vi "Fault_ID_Parse_FL24_Dryer.vi"(8 "Enum":enum16{"Sequence", "Table"}(ring), 11 "Numeric":u32) -> (3 "String":string)   [LabVIEW 2016]
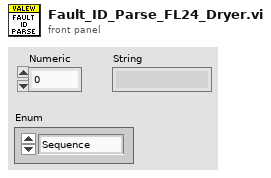
[diagram p1: front panel]
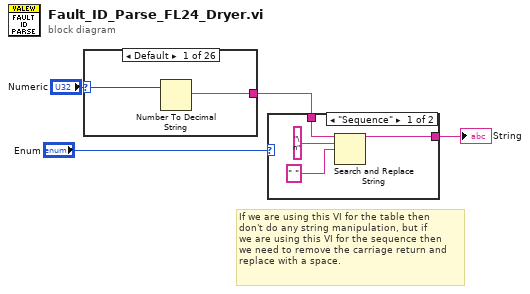
[diagram p0: block diagram]
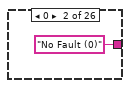
[diagram p3: hidden frame]
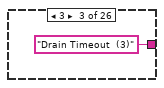
[diagram p4: hidden frame]
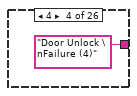
[diagram p5: hidden frame]
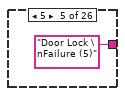
[diagram p6: hidden frame]
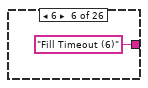
[diagram p7: hidden frame]
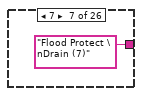
[diagram p8: hidden frame]
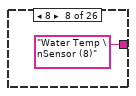
[diagram p9: hidden frame]
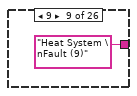
[diagram p10: hidden frame]
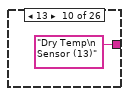
[diagram p11: hidden frame]
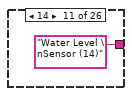
[diagram p12: hidden frame]
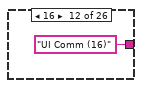
[diagram p13: hidden frame]
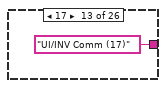
[diagram p14: hidden frame]
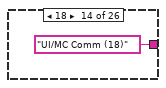
[diagram p15: hidden frame]
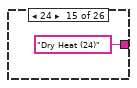
[diagram p16: hidden frame]
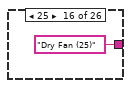
[diagram p17: hidden frame]
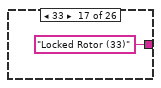
[diagram p18: hidden frame]
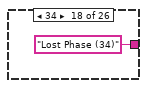
[diagram p19: hidden frame]
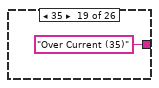
[diagram p20: hidden frame]
diagram:
  # "If we are using this VI for the table then\ndon't do any string manipulation, but if\nwe are using this VI for the sequence then\nwe need to remove the carriage return and\nreplace with a space."
  n1 = case shown="Default" "Numeric" {
    selector: "Numeric" -> [w6 _ _ _ _ _ _ _ _ _ _ _ _ _ _ _ _ _ _ _ _ _ _ _ _ _]
    tunnel: [w5 "No Fault (0)" "Drain Timeout  (3)" "Door Unlock \nFailure (4)" "Door Lock \nFailure (5)" "Fill Timeout (6)" "Flood Protect \nDrain (7)" "Water Temp \nSensor (8)" "Heat System \nFault (9)" "Dry Temp\n Sensor (13)" "Water Level \nSensor (14)" "UI Comm (16)" "UI/INV Comm (17)" "UI/MC Comm (18)" "Dry Heat (24)" "Dry Fan (25)" "Locked Rotor (33)" "Lost Phase (34)" "Over Current (35)" "Motor Current \nCircuit (36)" "Under \nVoltage (37)" "Motor \nOverheat (38)" "IMP Overheat (39)" "Drive Self \nCheck (40)" "MC Over \nVoltage (42)" "MC Check (43)"] -> w3
    frame Default {
      n2 = Number To Decimal String(number=w6) -> (decimal integer string=w5:string)  [unwired: 1 in]
    }
    frame 0 {
    }
    frame 3 {
    }
    frame 4 {
    }
    frame 5 {
    }
    frame 6 {
    }
    frame 7 {
    }
    frame 8 {
    }
    frame 9 {
    }
    frame 13 {
    }
    frame 14 {
    }
    frame 16 {
    }
    frame 17 {
    }
    frame 18 {
    }
    frame 24 {
    }
    frame 25 {
    }
    frame 33 {
    }
    frame 34 {
    }
    frame 35 {
    }
    frame 36 {
    }
    frame 37 {
    }
    frame 38 {
    }
    frame 39 {
    }
    frame 40 {
    }
    frame 42 {
    }
    frame 43 {
    }
  }
  n3 = case shown="\"Sequence\"" "Enum" {
    tunnel: w3 -> [w35 w36]
    tunnel: [w32 w36] -> w2
    frame "Sequence" {
      n4 = Search and Replace String(input string=w35, search string="\n", replace string=" " ("replace string (\"\")")) -> (result string=w32:string)  [unwired: 5 in, 3 out]
    }
    frame "Table" {
    }
  }
  "String" <- w2
